vi "LV Dev Doc - Instantiate with Path.vi"(0 "LV Doc Path":path, 11 "error in (no error)":errorcluster) -> (4 "LV DEV":refnum<class "LV DEV.lvclass">, 15 "error out":errorcluster)   [LabVIEW 2016, in "LV DEV.lvclass"]
uses:
  LV DEV.lvclass
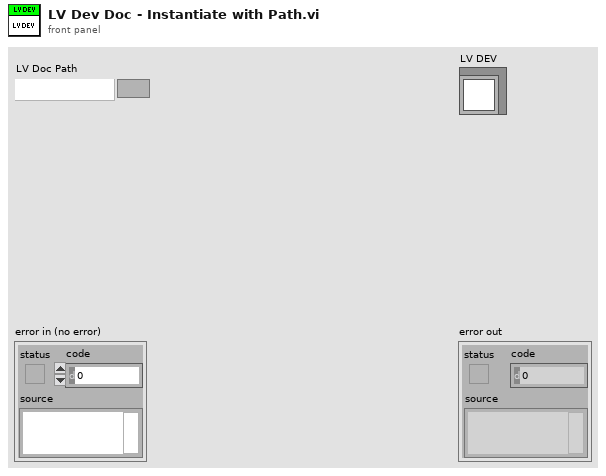
[diagram p1: front panel]
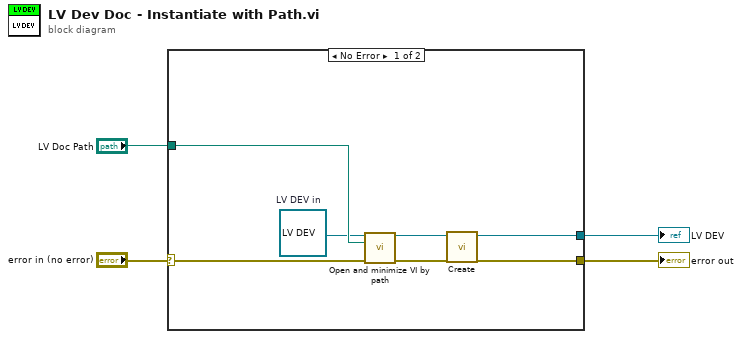
[diagram p0: block diagram]
diagram:
  n1 = case shown="No Error" "error in (no error)" {
    selector: "error in (no error)" -> [w11 w12]
    tunnel: [w7 w12] -> w3
    tunnel: "LV Doc Path" -> [w10 _]
    tunnel: [w8 _] -> w1
    frame No Error {
      w9 = refnum<class "LV DEV.lvclass"> refnum  # LV DEV in
      n2 = call "Open and minimize VI by path.vi"("LV DEV.lvclass"=w9, "Vi Path"=w10, "Error in"=w11) -> ("LV DEV.lvclass"=w6:refnum<class "LV DEV.lvclass">, "Error Out"=w5:errorcluster)  [unwired: 11 in]
      n3 = call-dynamic "Create.vi"("error in (no error)"=w5, "Document in"=w6) -> ("error out"=w7:errorcluster, "Document out"=w8:refnum<class "LV DEV.lvclass">)  [unwired: 8 in]
    }
    frame Error {
    }
  }
  "error out" <- w3
  "LV DEV" <- w1
